vi "switchmagnet_fpga.vi"() -> ()   [LabVIEW 2009]
uses:
  <vilib>/LabVIEW Targets/FPGA/cRIO/shared/nicrio_ModuleControls/nicrio_cRIO-9871_DataBitsEnum.ctl
  <vilib>/LabVIEW Targets/FPGA/cRIO/shared/nicrio_ModuleControls/nicrio_cRIO-9871_ParityEnum.ctl
  <vilib>/eio/EIOMethodNode/EIOMethodNode.xnode
  <vilib>/rvi/eio/nirviEIOMethodImplementation/nirviEIOMethodImplementation.xnode
  <vilib>/rvi/eio/common/nirviEmuTemplateMethod_errors.vi
  <vilib>/rvi/eio/common/nirviEmuClasses.ctl
  <vilib>/eio/EIOPropertyNode/EIOPropertyNode.xnode
  <vilib>/rvi/eio/nirviEIOPropertyImplementation/nirviEIOPropertyImplementation.xnode
  <vilib>/rvi/eio/common/nirviEmuTemplatePropertySet_noerrors.vi
panel:
  out "Numeric 4":i32
  out "Data":u8
  out "Timed Out":bool
  out "Numeric 2":i32
  out "Array":u8[](array[numeric])
  out "error out":errorcluster
  out "Numeric 3":i32
  in  "data 2":u8[](array[numeric])=[0, 0, 0, 0, 0, 0, 0, 0, 0, 0]
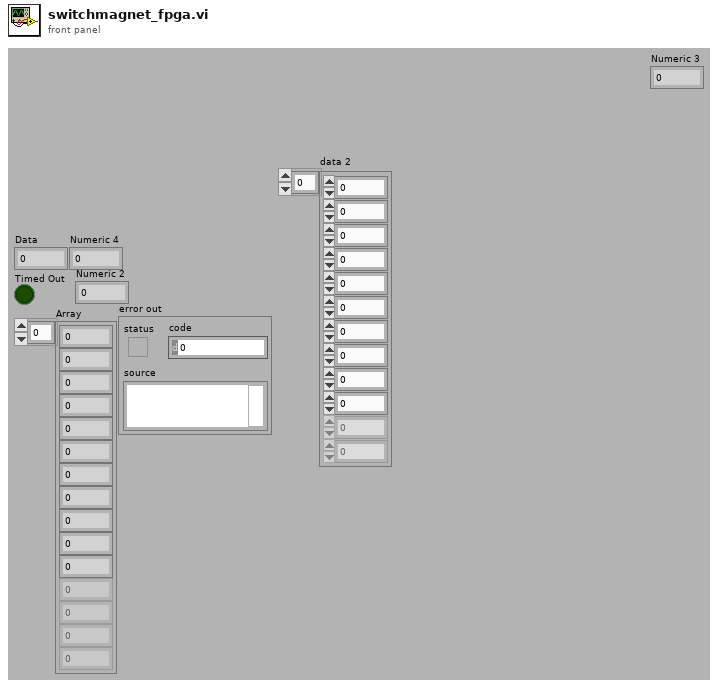
[diagram p1: front panel]
types:
  T1 = typedef "nicrio_cRIO-9871_ParityEnum.ctl" = enum8{"None", "Odd", "Even", "Mark", "Space"}
  T2 = typedef "nicrio_cRIO-9871_DataBitsEnum.ctl" = enum8{"5", "6", "7", "8"}
  T3 = typedef "nirviEmuClasses.ctl" = enum16{"IO Read", "IO Write", "Method", "Property Read", "Property Write"}
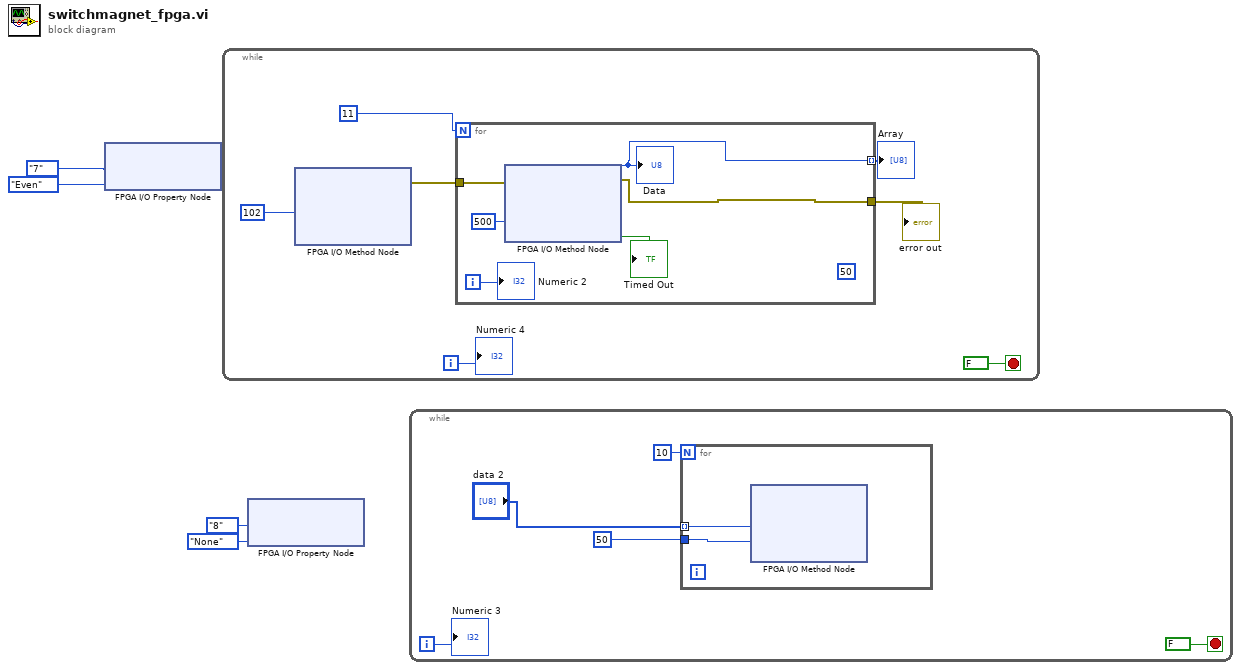
[diagram p0: block diagram]
diagram:
  n1 = xnode "FPGA I/O Property Node"("Data Bits"=nicrio_cRIO-9871_DataBitsEnum."7", "Parity"=nicrio_cRIO-9871_ParityEnum."Even") -> ()  [unwired: 1 in, 1 out]
  n2 = while {
    i -> [w10]
    stop <- FALSE stop-if-true
    w7 = u8 102 ("Data")
    n3 = xnode "FPGA I/O Method Node"("Data"=w7, "Timeout (ms)"=w7) -> ("error out"=w6:errorcluster)  [unwired: 2 in, 2 out]
    n4 = for {
      N: 11 ("Numeric 3") -> [_]
      tunnel: [w44] -> w8 mode=indexing
      tunnel: w6 -> [w42]
      tunnel: [w41] -> w5
      i -> [w43]
      (unwired) 50 ("Timeout")
      n5 = xnode "FPGA I/O Method Node"("error in"=w42, "Timeout (ms)"=500) -> ("error out"=w41:errorcluster, "Data"=w44:u8, "Timed Out"=→"Timed Out":bool)  [unwired: 1 in, 1 out]
      "Data" <- w44
      "Numeric 2" <- w43
    }
    "Array" <- w8
    "error out" <- w5
    "Numeric 4" <- w10
  }
  n6 = xnode "FPGA I/O Property Node"("Data Bits"=nicrio_cRIO-9871_DataBitsEnum."8", "Parity"=nicrio_cRIO-9871_ParityEnum."None") -> ()  [unwired: 1 in, 1 out]
  n7 = while {
    i -> [w87]
    stop <- FALSE stop-if-true
    n8 = for {
      N: 10 -> [_]
      tunnel: 50 ("Timeout (ms)") -> [w90]
      tunnel: "data 2" -> [w89] mode=indexing
      n9 = xnode "FPGA I/O Method Node"("Data"=w89, "Timeout (ms)"=w90) -> ()  [unwired: 2 in, 3 out]
    }
    "Numeric 3" <- w87
  }
